vi "create data to printer.vi"(11 "Data":T1) -> (0 "Print Barcode":string, 3 "Printer Data":string[](array[string]))   [LabVIEW 2015]
uses:
  Data base/database cluster.ctl
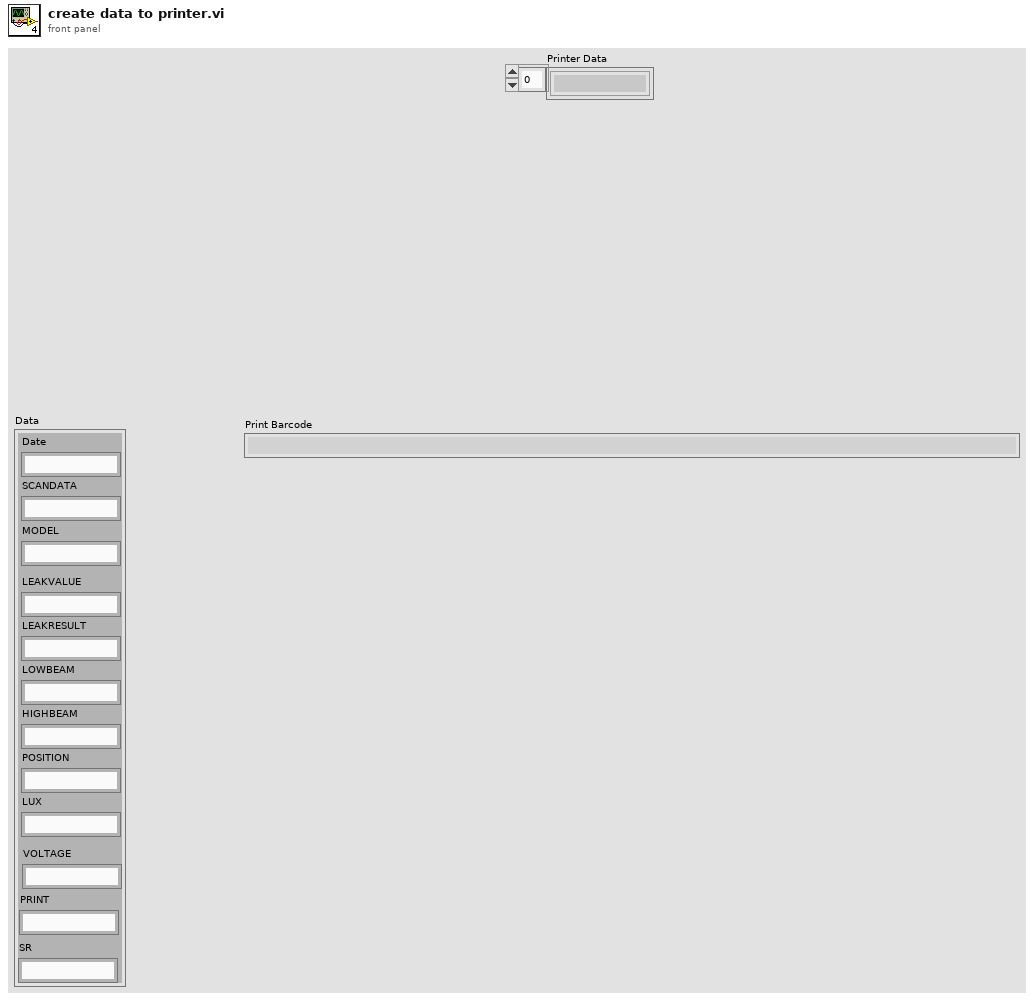
[diagram p1: front panel]
types:
  T1 = typedef "database cluster.ctl" = cluster{"Date":string, "SCANDATA":string, "MODEL":string, "LEAKVALUE":string, "LEAKRESULT":string, "LOWBEAM":string, "HIGHBEAM":string, "POSITION":string, "LUX":string, "VOLTAGE":string, "PRINT":string, "SR":string}
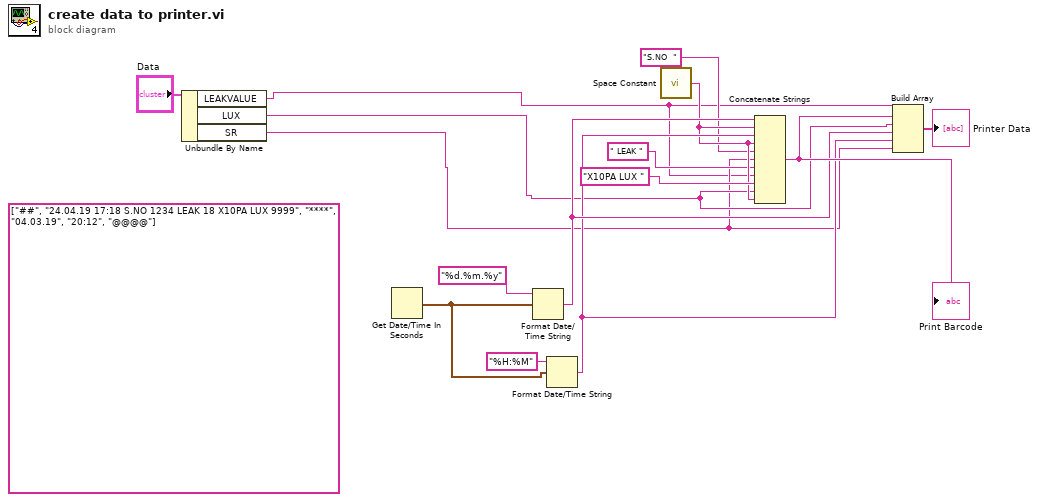
[diagram p0: block diagram]
diagram:
  (unwired) string[] ["##", "24.04.19 17:18 S.NO 1234 LEAK 18 X10PA LUX 9999", "****", "04.03.19", "20:12", "@@@@"] ("array 2")
  n1 = Unbundle By Name("Data") -> ("LEAKVALUE"=w1:string, "LUX"=w6:string, "SR"=w2:string)
  n2 = Get Date/Time In Seconds() -> (seconds since 1Jan1904=w13:timestamp)
  n3 = Format Date/Time String(time format string (%c)="%d.%m.%y", seconds (now)=w13) -> (date/time string=w10:string)  [unwired: 1 in]
  n4 = Format Date/Time String(time format string (%c)="%H:%M", seconds (now)=w13) -> (date/time string=w9:string)  [unwired: 1 in]
  n5 = call <vilib>:"Space Constant.vi"() -> ("String"=w8:string)
  n6 = Concatenate Strings(w10, w8, w9, w8, "S.NO  " ("time format string (%c)"), w2, " LEAK " ("time format string (%c)"), w1, "X10PA LUX " ("time format string (%c)"), w6, w8) -> (w12:string)
  "Print Barcode" <- w12
  n7 = Build Array(w1, w12, w6, w10, w9, w2) -> (→"Printer Data":string[])
